vi "Begin.vi"(11 "Image Size":T1=enum."320x240") -> (0 "error out":errorcluster)   [LabVIEW 2012]
doc: "Called before other user functions, this VI is expected to open initial I/O refnums, load in file data, and do all program initialization. Notice that the <B>error out</B> terminal is simply used for data flow. Wiring it to other structures or subVIs ensures that this VI runs first."
uses:
  <vilib>/Rock Robotics/WPI/Camera/WPI_CameraImageSize.ctl
  <vilib>/Rock Robotics/WPI/DriverStation/WPI_DriverStationRobotMode2.ctl
  <vilib>/Rock Robotics/SystemInterfaces/DIO/FPGA_DIOPWMChannel.ctl
  <vilib>/Rock Robotics/WPI/Joystick/WPI_JoystickDeviceEnum.ctl
  <vilib>/Rock Robotics/SystemInterfaces/Typedef/FPGA_TypedefDigitalModule.ctl
  <vilib>/Rock Robotics/WPI/Relay/WPI_RelayDirection.ctl
  <vilib>/Rock Robotics/SystemInterfaces/DIO/FPGA_DIORelayChannel.ctl
  <vilib>/Rock Robotics/SystemInterfaces/AI/FPGA_AIChannel.ctl
  <vilib>/Rock Robotics/SystemInterfaces/AI/FPGA_AIGyroChannel.ctl
  <vilib>/Rock Robotics/SystemInterfaces/DIO/FPGA_DIOChannel.ctl
  <vilib>/Rock Robotics/WPI/Camera/WPI_CameraFrameRate.ctl
  Robot Global Data.vi
  <vilib>/Rock Robotics/WPI/MotorControl/WPI_MotorControlOpen Victor.vi
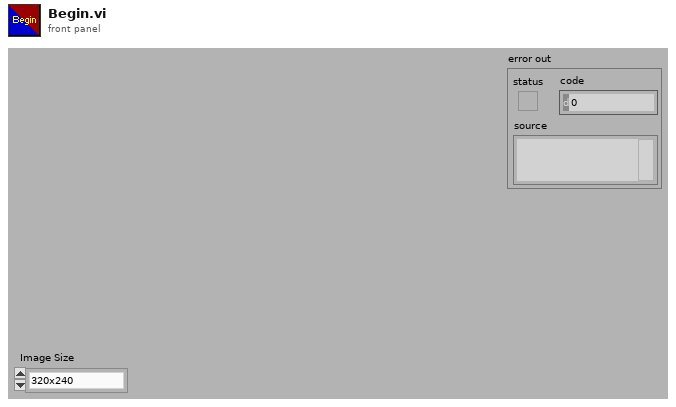
[diagram p1: front panel]
types:
  T1 = typedef "WPI_CameraImageSize.ctl" = enum16{"640x480", "320x240", "160x120"}
  T2 = typedef "FPGA_DIORelayChannel.ctl" = enum8{"Relay 1", "Relay 2", "Relay 3", "Relay 4", "Relay 5", "Relay 6", "Relay 7", "Relay 8", "Invalid"}
  T3 = typedef "WPI_RelayDirection.ctl" = enum16{"Both directions", "Forward only", "Reverse only"}
  T4 = typedef "WPI_CameraFrameRate.ctl" = u32
  T5 = typedef "FPGA_AIChannel.ctl" = enum8{"AI 1", "AI 2", "AI 3", "AI 4", "AI 5", "AI 6", "AI 7", "AI 8", "Invalid"}
  T6 = typedef "FPGA_DIOChannel.ctl" = enum8{"DIO 1", "DIO 2", "DIO 3", "DIO 4", "DIO 5", "DIO 6", "DIO 7", "DIO 8", "DIO 9", "DIO 10", "DIO 11", "DIO 12", "DIO 13", "DIO 14", "Invalid"}
  T7 = typedef "FPGA_TypedefDigitalModule.ctl" = enum16{"Digital Module 1", "Digital Module 2"}
  T8 = typedef "FPGA_DIOPWMChannel.ctl" = enum8{"PWM 1", "PWM 2", "PWM 3", "PWM 4", "PWM 5", "PWM 6", "PWM 7", "PWM 8", "PWM 9", "PWM 10", "Invalid"}
  T9 = typedef "FPGA_AIGyroChannel.ctl" = enum8{"AI 1", "AI 2", "Invalid"}
  T10 = typedef "WPI_JoystickDeviceEnum.ctl" = enum16{"USB 1", "USB 2", "USB 3", "USB 4", "Kinect 1", "Kinect 2"}
  T11 = typedef "WPI_DriverStationRobotMode2.ctl" = enum16{"Autonomous Disabled", "Autonomous Enabled", "Teleop Disabled", "Teleop Enabled", "Timeout", "Finish", "Test Disabled", "Test Enabled"}
  T12 = typedef "WPI_MotorControlDeviceRef.ctl" = cluster{"DeviceStatus":errorcluster, "Type":enum16{"PWM", "CAN"}, "PWM":cluster{"Digital Module":T7, "PWM Channel":T8, "DeadBand":T13}, "CAN":cluster{"Device Number":u8, "Control Mode":T14, "Semaphore":T15, "Max Vout":dbl}, "Invert":bool, "TransformRef":T16, "InvTransformRef":T16}
  T13 = typedef "WPI_PWMDeadband.ctl" = cluster{"Name":string, "maxPositivePwm":i32, "minPositivePwm":i32, "centerPwm":i32, "maxNegativePwm":i32, "minNegativePwm":i32, "angularRange":u16}
  T14 = typedef "WPI_CANJaguar_ControlMode.ctl" = enum8{"Percent VBus", "Current", "Speed", "Position", "Voltage"}
  T15 = typedef "Semaphore RefNum" = refnum<k1>
  T16 = typedef "WPI_PWMTransform_ConPane.ctl" = refnum<vi>
  T17 = typedef "WPI_CameraDevRef.ctl" = cluster{"Camera Address":string, "CameraStatus":errorcluster, "Acquire Image Notifier":refnum<notifier>}
  T18 = typedef "WPI_JoystickDevRef.ctl" = cluster{"Device":T10}
  T19 = typedef "WPI_ServoDeviceRef.ctl" = cluster{"DeviceStatus":errorcluster, "Digital Module":T7, "PWM Channel":T8, "DeadBand":T13}
  T20 = typedef "WPI_DigitalInputDevRef.ctl" = cluster{"DevStatus":errorcluster, "DIO Channel":T6, "Digital Module":T7}
  T21 = typedef "WPI_RelayDevRef.ctl" = cluster{"DevStatus":errorcluster, "Relay Channel":T2, "Digital Module":T7, "Relay Direction":T3}
  T22 = typedef "WPI_AnalogChannelDevRef.ctl" = cluster{"DevStatus":errorcluster, "Analog Module":T23, "Analog Channel":T5}
  T23 = typedef "FPGA_TypedefAnalogModule.ctl" = enum16{"Analog Module 1", "Analog Module 2"}
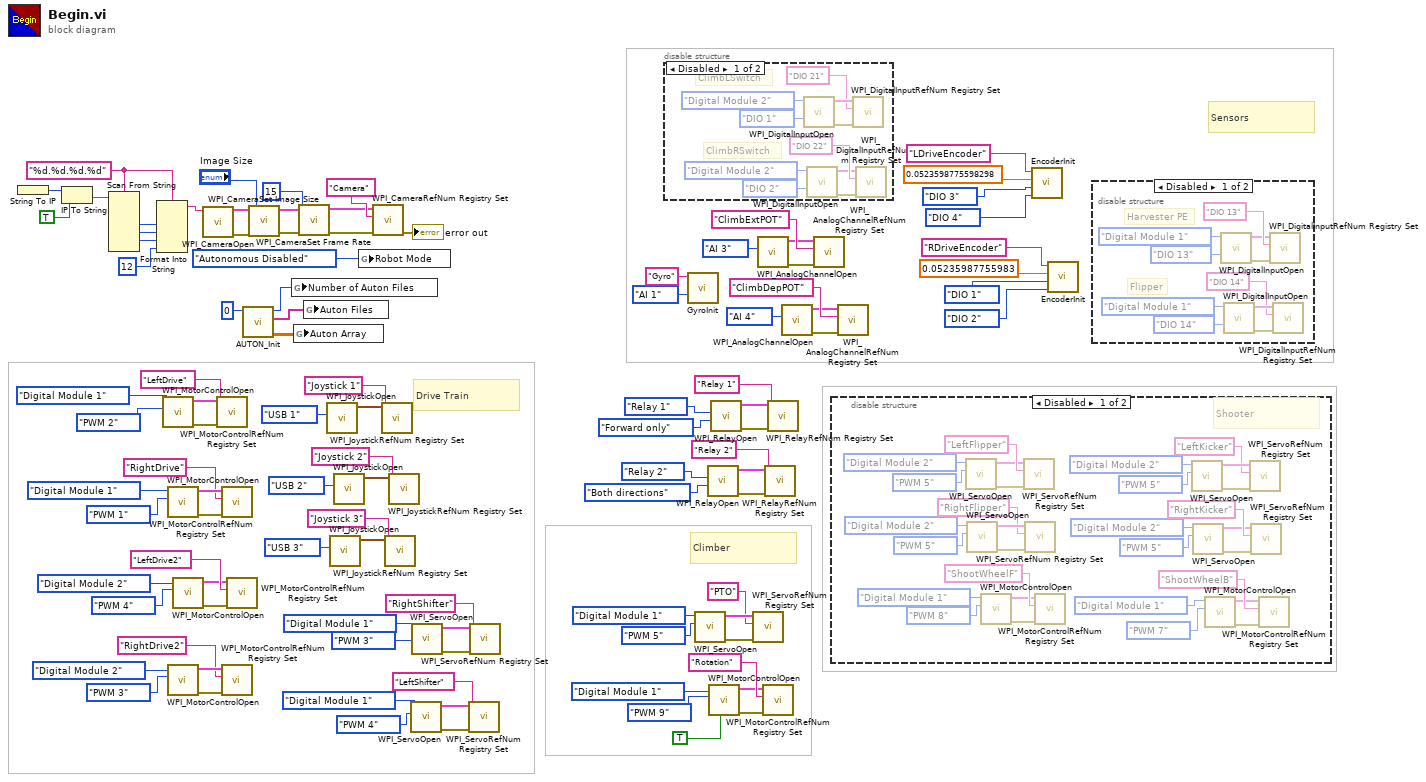
[diagram p0: block diagram]
diagram:
  w15 = "%d.%d.%d.%d" ("format string")
  # "Drive Train"
  # "Climber"
  # "Sensors"
  n1 = String To IP() -> (0:w22:u32)  [unwired: 1 in]
  n2 = IP To String(1:TRUE ("dot notation? (F)"), 2:w22) -> (0:w20:string)
  n3 = Scan From String(format string=w15, input string=w20) -> (output 1=w19:i32, output 2=w18:i32, output 3=w17:i32)  [unwired: 7 in, 3 out]
  n4 = Format Into String(format string=w15, w19, w18, w17, 12 ("Compression")) -> (resulting string=w14:string)  [unwired: 2 in, 1 out]
  n5 = call-poly <vilib>:"WPI_MotorControlOpen.vi"("PWM Channel"=FPGA_DIOPWMChannel."PWM 2", "Digital Module (Module 1)"=FPGA_TypedefDigitalModule."Digital Module 1") -> ("error out"=w90:errorcluster, "MotorControlDeviceRef"=w91:T12)  [unwired: 8 in]
  n6 = call-poly <vilib>:"WPI_MotorControlOpen.vi"("PWM Channel"=FPGA_DIOPWMChannel."PWM 1", "Digital Module (Module 1)"=FPGA_TypedefDigitalModule."Digital Module 1") -> ("error out"=w97:errorcluster, "MotorControlDeviceRef"=w96:T12)  [unwired: 8 in]
  n7 = call-poly <vilib>:"WPI_MotorControlOpen.vi"("PWM Channel"=FPGA_DIOPWMChannel."PWM 3", "Digital Module (Module 1)"=FPGA_TypedefDigitalModule."Digital Module 2") -> ("error out"=w79:errorcluster, "MotorControlDeviceRef"=w78:T12)  [unwired: 8 in]
  n8 = call-poly <vilib>:"WPI_MotorControlOpen.vi"("PWM Channel"=FPGA_DIOPWMChannel."PWM 4", "Digital Module (Module 1)"=FPGA_TypedefDigitalModule."Digital Module 2") -> ("error out"=w70:errorcluster, "MotorControlDeviceRef"=w71:T12)  [unwired: 8 in]
  n9 = call <vilib>:"WPI_CameraOpen.vi"("Camera Address"=w14) -> ("error out"=w13:errorcluster, "CameraDevRef"=w12:T17)  [unwired: 1 in, 8 out]
  n10 = call <vilib>:"WPI_MotorControlRefNum Registry Set.vi"("error in (no error)"=w90, "refnum name"="LeftDrive", "MotorControlDevRef"=w91) -> ()  [unwired: 7 in, 2 out]
  n11 = call <vilib>:"WPI_MotorControlRefNum Registry Set.vi"("error in (no error)"=w97, "refnum name"="RightDrive", "MotorControlDevRef"=w96) -> ()  [unwired: 7 in, 2 out]
  n12 = call <vilib>:"WPI_MotorControlRefNum Registry Set.vi"("error in (no error)"=w79, "refnum name"="RightDrive2", "MotorControlDevRef"=w78) -> ()  [unwired: 7 in, 2 out]
  n13 = call <vilib>:"WPI_MotorControlRefNum Registry Set.vi"("error in (no error)"=w70, "refnum name"="LeftDrive2", "MotorControlDevRef"=w71) -> ()  [unwired: 7 in, 2 out]
  n14 = call "AUTON_Init.vi"("Default File"=0) -> ("Auton Array"=w98:dbl[][], "Auton Files"=w99:string[], "Number of Auton Files"=w100:i64)  [unwired: 8 in]
  n15 = call <vilib>:"WPI_CameraSet Image Size.vi"("error in (no error)"=w13, "Image Size"="Image Size", "CameraDevRef"=w12) -> ("error out"=w10:errorcluster, "CameraDevRef Out"=w11:T17)  [unwired: 7 out]
  n16 = global write "Robot Global Data.vi" "Number of Auton Files"(w100) -> ()
  n17 = global write "Robot Global Data.vi" "Auton Array"(w98) -> ()
  n18 = call <vilib>:"WPI_CameraSet Frame Rate.vi"("error in (no error)"=w10, "Frame Rate (fps)"=T4 15, "CameraDevRef"=w11) -> ("error out"=w9:errorcluster, "CameraDevRef Out"=w8:T17)  [unwired: 7 out]
  n19 = global write "Robot Global Data.vi" "Auton Files"(w99) -> ()
  n20 = call <vilib>:"WPI_JoystickOpen.vi"("JoystickDevice"=WPI_JoystickDeviceEnum."USB 1") -> ("JoystickDevRef"=w81:T18)  [unwired: 10 in]
  n21 = call <vilib>:"WPI_JoystickOpen.vi"("JoystickDevice"=WPI_JoystickDeviceEnum."USB 3") -> ("JoystickDevRef"=w87:T18)  [unwired: 10 in]
  n22 = call <vilib>:"WPI_JoystickOpen.vi"("JoystickDevice"=WPI_JoystickDeviceEnum."USB 2") -> ("JoystickDevRef"=w86:T18)  [unwired: 10 in]
  n23 = global write "Robot Global Data.vi" "Robot Mode"(WPI_DriverStationRobotMode2."Autonomous Disabled" ("Robot Mode")) -> ()
  n24 = call <vilib>:"WPI_CameraRefNum Registry Set.vi"("error in (no error)"=w9, "refnum name"="Camera", "CameraDevRef"=w8) -> ("error out"=→"error out":errorcluster)  [unwired: 8 out]
  n25 = call <vilib>:"WPI_JoystickRefNum Registry Set.vi"("refnum name"="Joystick 1", "JoystickDevRef"=w81) -> ()  [unwired: 8 in, 2 out]
  n26 = call <vilib>:"WPI_JoystickRefNum Registry Set.vi"("refnum name"="Joystick 3", "JoystickDevRef"=w87) -> ()  [unwired: 8 in, 2 out]
  n27 = call <vilib>:"WPI_JoystickRefNum Registry Set.vi"("refnum name"="Joystick 2", "JoystickDevRef"=w86) -> ()  [unwired: 8 in, 2 out]
  n28 = call <vilib>:"WPI_ServoOpen.vi"("PWM Channel"=FPGA_DIOPWMChannel."PWM 4", "Digital Module (Module 1)"=FPGA_TypedefDigitalModule."Digital Module 1") -> ("error out"=w63:errorcluster, "ServoDeviceRef"=w56:T19)  [unwired: 8 in]
  n29 = call <vilib>:"WPI_ServoOpen.vi"("PWM Channel"=FPGA_DIOPWMChannel."PWM 3", "Digital Module (Module 1)"=FPGA_TypedefDigitalModule."Digital Module 1") -> ("error out"=w62:errorcluster, "ServoDeviceRef"=w61:T19)  [unwired: 8 in]
  n30 = call <vilib>:"WPI_ServoRefNum Registry Set.vi"("error in (no error)"=w63, "refnum name"="LeftShifter", "ServoDeviceRef"=w56) -> ()  [unwired: 7 in, 2 out]
  n31 = call <vilib>:"WPI_ServoRefNum Registry Set.vi"("error in (no error)"=w62, "refnum name"="RightShifter", "ServoDeviceRef"=w61) -> ()  [unwired: 7 in, 2 out]
  n32 = disable-structure shown="Disabled" {
    frame Disabled {
      # "ClimbRSwitch"
      # "ClimbLSwitch"
      n33 = call <vilib>:"WPI_DigitalInputOpen.vi"("DIO Channel"=FPGA_DIOChannel."DIO 1", "Digital Module (Module 1)"=FPGA_TypedefDigitalModule."Digital Module 2") -> ("error out"=w104:errorcluster, "DigitalInputDevRef"=w105:T20)  [unwired: 8 in]
      n34 = call <vilib>:"WPI_DigitalInputOpen.vi"("DIO Channel"=FPGA_DIOChannel."DIO 2", "Digital Module (Module 1)"=FPGA_TypedefDigitalModule."Digital Module 2") -> ("error out"=w111:errorcluster, "DigitalInputDevRef"=w110:T20)  [unwired: 8 in]
      n35 = call <vilib>:"WPI_DigitalInputRefNum Registry Set.vi"("error in (no error)"=w104, "refnum name"="DIO 21", "DigitalInputDevRef"=w105) -> ()  [unwired: 7 in, 2 out]
      n36 = call <vilib>:"WPI_DigitalInputRefNum Registry Set.vi"("error in (no error)"=w111, "refnum name"="DIO 22", "DigitalInputDevRef"=w110) -> ()  [unwired: 7 in, 2 out]
    }
    frame Enabled {
    }
  }
  n37 = call "GyroInit.vi"("refnum name"="Gyro", "Analog Channel"=FPGA_AIGyroChannel."AI 1") -> ()  [unwired: 8 in]
  n38 = call <vilib>:"WPI_ServoOpen.vi"("PWM Channel"=FPGA_DIOPWMChannel."PWM 5", "Digital Module (Module 1)"=FPGA_TypedefDigitalModule."Digital Module 1") -> ("error out"=w41:errorcluster, "ServoDeviceRef"=w40:T19)  [unwired: 8 in]
  n39 = call <vilib>:"WPI_RelayOpen.vi"("Relay Direction"=WPI_RelayDirection."Both directions", "Relay Channel"=FPGA_DIORelayChannel."Relay 2") -> ("error out"=w64:errorcluster, "RelayDevRef"=w65:T21)  [unwired: 8 in]
  n40 = call-poly <vilib>:"WPI_MotorControlOpen.vi"("Invert"=TRUE, "PWM Channel"=FPGA_DIOPWMChannel."PWM 9", "Digital Module (Module 1)"=FPGA_TypedefDigitalModule."Digital Module 1") -> ("error out"=w46:errorcluster, "MotorControlDeviceRef"=w45:T12)  [unwired: 7 in]
  n41 = call <vilib>:"WPI_RelayOpen.vi"("Relay Direction"=WPI_RelayDirection."Forward only", "Relay Channel"=FPGA_DIORelayChannel."Relay 1") -> ("error out"=w5:errorcluster, "RelayDevRef"=w4:T21)  [unwired: 8 in]
  n42 = call <vilib>:"WPI_ServoRefNum Registry Set.vi"("error in (no error)"=w41, "refnum name"="PTO", "ServoDeviceRef"=w40) -> ()  [unwired: 7 in, 2 out]
  n43 = call <vilib>:"WPI_AnalogChannelOpen.vi"("Analog Channel"=FPGA_AIChannel."AI 3") -> ("error out"=w25:errorcluster, "AIDeviceRef"=w26:T22)  [unwired: 9 in]
  n44 = call <vilib>:"WPI_MotorControlRefNum Registry Set.vi"("error in (no error)"=w46, "refnum name"="Rotation", "MotorControlDevRef"=w45) -> ()  [unwired: 7 in, 2 out]
  n45 = call <vilib>:"WPI_RelayRefNum Registry Set.vi"("error in (no error)"=w64, "refnum name"="Relay 2", "RelayDevRef"=w65) -> ()  [unwired: 7 in, 2 out]
  n46 = call <vilib>:"WPI_RelayRefNum Registry Set.vi"("error in (no error)"=w5, "refnum name"="Relay 1", "RelayDevRef"=w4) -> ()  [unwired: 7 in, 2 out]
  n47 = call <vilib>:"WPI_AnalogChannelOpen.vi"("Analog Channel"=FPGA_AIChannel."AI 4") -> ("error out"=w50:errorcluster, "AIDeviceRef"=w51:T22)  [unwired: 9 in]
  n48 = call <vilib>:"WPI_AnalogChannelRefNum Registry Set.vi"("error in (no error)"=w25, "refnum name"="ClimbExtPOT", "AIDeviceRef"=w26) -> ()  [unwired: 7 in, 2 out]
  n49 = disable-structure shown="Disabled" {
    frame Disabled {
      # "Shooter"
      n50 = call <vilib>:"WPI_ServoOpen.vi"("PWM Channel"=FPGA_DIOPWMChannel."PWM 5", "Digital Module (Module 1)"=FPGA_TypedefDigitalModule."Digital Module 2") -> ("error out"=w128:errorcluster, "ServoDeviceRef"=w129:T19)  [unwired: 8 in]
      n51 = call <vilib>:"WPI_ServoOpen.vi"("PWM Channel"=FPGA_DIOPWMChannel."PWM 5", "Digital Module (Module 1)"=FPGA_TypedefDigitalModule."Digital Module 2") -> ("error out"=w127:errorcluster, "ServoDeviceRef"=w126:T19)  [unwired: 8 in]
      n52 = call-poly <vilib>:"WPI_MotorControlOpen.vi"("PWM Channel"=FPGA_DIOPWMChannel."PWM 8", "Digital Module (Module 1)"=FPGA_TypedefDigitalModule."Digital Module 1") -> ("error out"=w139:errorcluster, "MotorControlDeviceRef"=w140:T12)  [unwired: 8 in]
      n53 = call <vilib>:"WPI_ServoRefNum Registry Set.vi"("error in (no error)"=w128, "refnum name"="LeftFlipper", "ServoDeviceRef"=w129) -> ()  [unwired: 7 in, 2 out]
      n54 = call <vilib>:"WPI_ServoRefNum Registry Set.vi"("error in (no error)"=w127, "refnum name"="RightFlipper", "ServoDeviceRef"=w126) -> ()  [unwired: 7 in, 2 out]
      n55 = call <vilib>:"WPI_MotorControlRefNum Registry Set.vi"("error in (no error)"=w139, "refnum name"="ShootWheelF", "MotorControlDevRef"=w140) -> ()  [unwired: 7 in, 2 out]
      n56 = call <vilib>:"WPI_ServoOpen.vi"("PWM Channel"=FPGA_DIOPWMChannel."PWM 5", "Digital Module (Module 1)"=FPGA_TypedefDigitalModule."Digital Module 2") -> ("error out"=w118:errorcluster, "ServoDeviceRef"=w117:T19)  [unwired: 8 in]
      n57 = call <vilib>:"WPI_ServoOpen.vi"("PWM Channel"=FPGA_DIOPWMChannel."PWM 5", "Digital Module (Module 1)"=FPGA_TypedefDigitalModule."Digital Module 2") -> ("error out"=w113:errorcluster, "ServoDeviceRef"=w119:T19)  [unwired: 8 in]
      n58 = call-poly <vilib>:"WPI_MotorControlOpen.vi"("PWM Channel"=FPGA_DIOPWMChannel."PWM 7", "Digital Module (Module 1)"=FPGA_TypedefDigitalModule."Digital Module 1") -> ("error out"=w135:errorcluster, "MotorControlDeviceRef"=w134:T12)  [unwired: 8 in]
      n59 = call <vilib>:"WPI_ServoRefNum Registry Set.vi"("error in (no error)"=w118, "refnum name"="LeftKicker", "ServoDeviceRef"=w117) -> ()  [unwired: 7 in, 2 out]
      n60 = call <vilib>:"WPI_ServoRefNum Registry Set.vi"("error in (no error)"=w113, "refnum name"="RightKicker", "ServoDeviceRef"=w119) -> ()  [unwired: 7 in, 2 out]
      n61 = call <vilib>:"WPI_MotorControlRefNum Registry Set.vi"("error in (no error)"=w135, "refnum name"="ShootWheelB", "MotorControlDevRef"=w134) -> ()  [unwired: 7 in, 2 out]
    }
    frame Enabled {
    }
  }
  n62 = call <vilib>:"WPI_AnalogChannelRefNum Registry Set.vi"("error in (no error)"=w50, "refnum name"="ClimbDepPOT", "AIDeviceRef"=w51) -> ()  [unwired: 7 in, 2 out]
  n63 = call "EncoderInit.vi"("refnum name"="LDriveEncoder", "DistancePerCount"=0.0523598775598298, "DIO Channel"=FPGA_DIOChannel."DIO 3", "DIO Channel 2"=FPGA_DIOChannel."DIO 4") -> ()  [unwired: 7 in]
  n64 = call "EncoderInit.vi"("refnum name"="RDriveEncoder", "DistancePerCount"=0.05235987755983, "DIO Channel"=FPGA_DIOChannel."DIO 1", "DIO Channel 2"=FPGA_DIOChannel."DIO 2") -> ()  [unwired: 7 in]
  n65 = disable-structure shown="Disabled" {
    frame Disabled {
      # "Flipper"
      # "Harvester PE"
      n66 = call <vilib>:"WPI_DigitalInputOpen.vi"("DIO Channel"=FPGA_DIOChannel."DIO 13", "Digital Module (Module 1)"=FPGA_TypedefDigitalModule."Digital Module 1") -> ("error out"=w151:errorcluster, "DigitalInputDevRef"=w150:T20)  [unwired: 8 in]
      n67 = call <vilib>:"WPI_DigitalInputOpen.vi"("DIO Channel"=FPGA_DIOChannel."DIO 14", "Digital Module (Module 1)"=FPGA_TypedefDigitalModule."Digital Module 1") -> ("error out"=w144:errorcluster, "DigitalInputDevRef"=w145:T20)  [unwired: 8 in]
      n68 = call <vilib>:"WPI_DigitalInputRefNum Registry Set.vi"("error in (no error)"=w151, "refnum name"="DIO 13", "DigitalInputDevRef"=w150) -> ()  [unwired: 7 in, 2 out]
      n69 = call <vilib>:"WPI_DigitalInputRefNum Registry Set.vi"("error in (no error)"=w144, "refnum name"="DIO 14", "DigitalInputDevRef"=w145) -> ()  [unwired: 7 in, 2 out]
    }
    frame Enabled {
    }
  }
